vi "Actuadores.vi"() -> ()   [LabVIEW 2017]
panel:
  out "Actuadores":T1
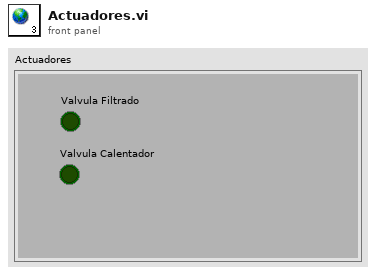
[diagram p1: front panel]
types:
  T1 = cluster{"Valvula Filtrado":bool, "Valvula Calentador":bool}
diagram:
